vi "TSM SSC Digital Configure Time Set Compare Edge.vi"(0 "Digital TSM In":T1, 5 "time set":string caption="Time Set", 7 "Compare Strobe (s)":dbl, 11 "error in":errorcluster) -> (4 "Digital TSM Out":T1, 15 "error out":errorcluster)   [LabVIEW 2020]
doc: "Configures the strobe edge time for the specified pins. Use this function to modify time set values after applying a timing sheet with the niDigital Apply Levels and Timing VI, or to create time sets programmatically without the use of timing sheets. This function does not modify the timing sheet file or the timing sheet contents that will be used in future calls to niDigital Apply Levels and Timing; it only affects the values of the current timing context."
uses:
  TSM/TSM SSC Digital.ctl
  <vilib>/NI_TestStand_SemiconductorModule/NI_TestStand_Semiconductor_Module.lvlibp/PinMap/Digital Pattern/PinQueryContext/DigitalPatternPinQueryContext.lvclass
  SSC Digital/SSC Digital.ctl
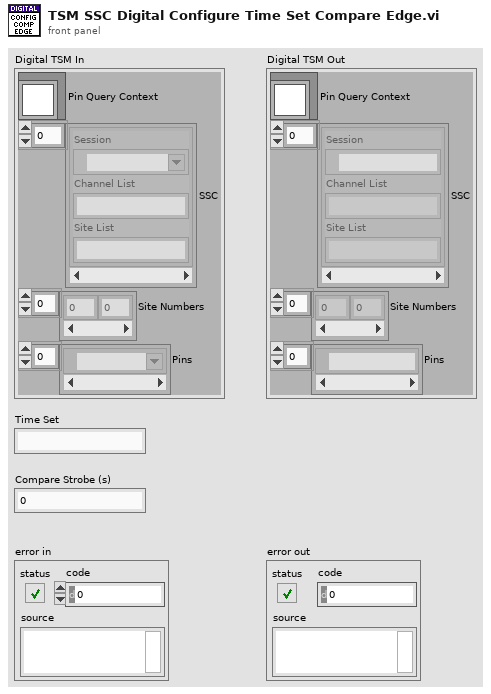
[diagram p1: front panel]
types:
  T1 = typedef "TSM SSC Digital.ctl" = cluster{"Pin Query Context":refnum<class "DigitalPatternPinQueryContext.lvclass">, "SSC":T2[], "Site Numbers":i32[], "Pins":tag[]}
  T2 = typedef "SSC Digital.ctl" = cluster{"Session":refnum<k15>, "Channel List":string, "Site List":string}
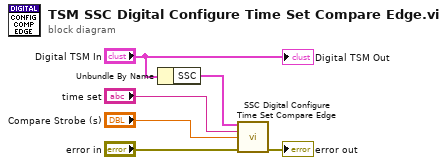
[diagram p0: block diagram]
diagram:
  n1 = Unbundle By Name("Digital TSM In") -> ("SSC"=w5:T2[])
  n2 = call "SSC Digital Configure Time Set Compare Edge.vi"("Digital SSC in"=w5, "time set"="time set", "Compare Strobe (s)"="Compare Strobe (s)", "error in"="error in") -> ("error out"=→"error out":errorcluster)  [unwired: 10 in, 1 out]
  "Digital TSM Out" <- "Digital TSM In"
